vi "Create Bus.vi"(8 "error in (no error)":errorcluster, 11 "Bus in":refnum<class "Bus.lvclass">) -> (0 "error out":errorcluster, 3 "Bus out":refnum<class "Bus.lvclass">)   [LabVIEW 2015, in "Bus.lvclass"]
uses:
  Bus.lvclass
  <vilib>/LIEF/Forms/Shape/Shape.lvclass/Shape.ctl
  <vilib>/LIEF/Forms/Line/Line.lvclass/Line.ctl
  <vilib>/LIEF/Forms/Shape/Write Selectable.vi
  <vilib>/LIEF/Forms/Shape/Write Movable.vi
  <vilib>/LIEF/Forms/Line/Write Style.vi
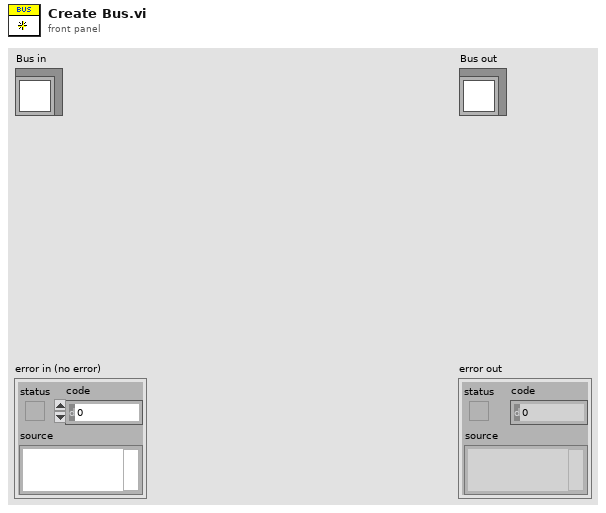
[diagram p1: front panel]
types:
  T1 = cluster{"Width":u16, "Style":enum32{"Solid", "Dash", "Dot", "DashDot", "DashDotDot"}}
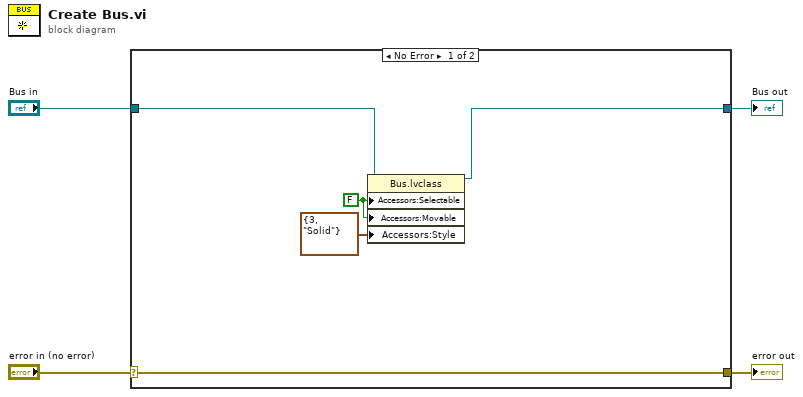
[diagram p0: block diagram]
diagram:
  n1 = case shown="No Error" "error in (no error)" {
    selector: "error in (no error)" -> [w9 w11]
    tunnel: [w9 w11] -> w3
    tunnel: [w7 w10] -> w1
    tunnel: "Bus in" -> [w8 w10]
    frame No Error {
      w6 = FALSE ("Selectable")
      n2 = property class="Bus.lvclass"(reference=w8, "Accessors:Selectable"=w6, "Accessors:Movable"=w6, "Accessors:Style"=T1 {"Width"=3, "Style"=enum."Solid"} ("Style")) -> (reference out=w7:refnum<class "Bus.lvclass">)  [unwired: 1 in, 1 out]
    }
    frame Error {
    }
  }
  "error out" <- w3
  "Bus out" <- w1
